vi "Exit.vi"(8 "error in (no error)":errorcluster, 11 "Old State":refnum<class "Command States.lvclass">) -> (0 "error out":errorcluster, 3 "New State":refnum<class "Command States.lvclass">)   [LabVIEW 2013, in "Command Actor.lvlib" / "Command States.lvclass"]
doc: "This is an abstract method. Override this method to define the behavior when you leave the state."
uses:
  Command States.lvclass
  Command/State Status.ctl
  <vilib>/ni/Actors/State Actor/State Actor/State Actor.lvclass
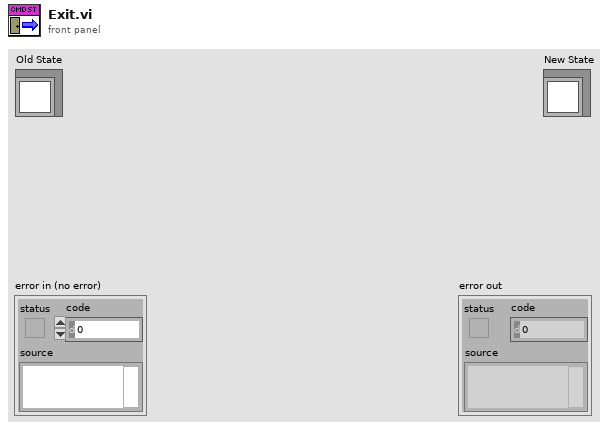
[diagram p1: front panel]
types:
  T1 = typedef "Command Actor.lvlib/Command States.lvclass/State Status.ctl" = cluster{"State Name":string, "State Entry Time":timestamp, "State Exit Time":timestamp}
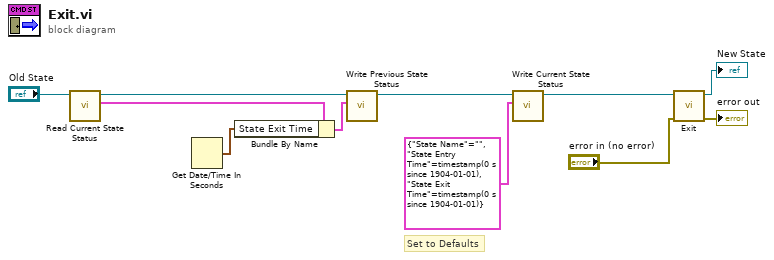
[diagram p0: block diagram]
diagram:
  # "Set to Defaults"
  n1 = call-dynamic "Read Current State Status.vi"("Command States in"="Old State") -> ("State Status"=w6:T1, "Command States out"=w7:refnum<class "Command States.lvclass">)  [unwired: 8 in, 1 out]
  n2 = Get Date/Time In Seconds() -> (seconds since 1Jan1904=w4:timestamp)
  n3 = Bundle By Name(cluster=w6, "State Exit Time"=w4) -> (w5:T1)
  n4 = call-dynamic "Write Previous State Status.vi"("State Status"=w5, "Command States in"=w7) -> ("Command States out"=w3:refnum<class "Command States.lvclass">)  [unwired: 8 in, 1 out]
  n5 = call-dynamic "Write Current State Status.vi"("State Status"=T1 {"State Name"="", "State Entry Time"=timestamp(0 s since 1904-01-01), "State Exit Time"=timestamp(0 s since 1904-01-01)}, "Command States in"=w3) -> ("Command States out"=w2:refnum<class "Command States.lvclass">)  [unwired: 8 in, 1 out]
  n6 = call-parent "Exit.vi"("error in (no error)"="error in (no error)", "Old State"=w2) -> ("error out"=→"error out":errorcluster, "New State"=→"New State":refnum<class "Command States.lvclass">)  [unwired: 8 in]
